vi "SPI_Close_Device.vi"(1 "Handle":u32) -> (0 "FTC_Status":u32)   [LabVIEW 2010]
uses:
  WINNT/system32/FTCSPI.dll
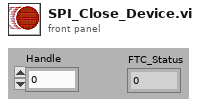
[diagram p1: front panel]
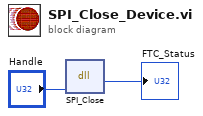
[diagram p0: block diagram]
diagram:
  n1 = dll-call lib="C:/Users/WINNT/system32/FTCSPI.dll" fn="SPI_Close"("Handle"="Handle") -> ("FTC_Status"=→"FTC_Status":u32)  [unwired: 4 in, 2 out]
